vi "4.5.vi"() -> ()   [LabVIEW 2017]
panel:
  out "循环执行的次数":dbl
  in  "指定值":dbl
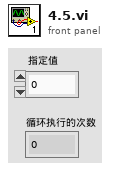
[diagram p1: front panel]
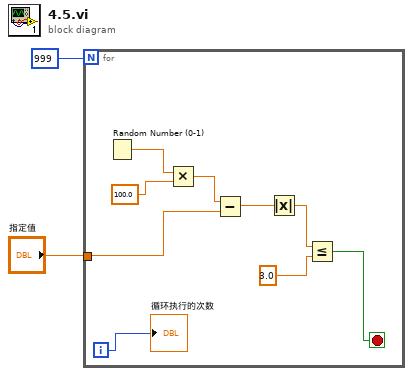
[diagram p0: block diagram]
diagram:
  n1 = for {
    N: 999 -> [_]
    tunnel: "指定值" -> [w7]
    i -> [w11]
    stop <- w3 stop-if-true
    n2 = Random Number (0-1)() -> (number: 0 to 1=w10:dbl)
    n3 = Multiply(x=w10, y=100.0) -> (x*y=w8:dbl)
    n4 = Subtract(x=w8, y=w7) -> (x-y=w6:dbl)
    n5 = Absolute Value(x=w6) -> (abs(x)=w5:dbl)
    n6 = Less Or Equal?(x=w5, y=3.0) -> (x <= y?=w3:bool)
    "循环执行的次数" <- w11
  }
